vi "Wash - Activate LED.vi"(8 "error in (no error)":errorcluster, 11 "View Model":T2) -> (0 "error out":errorcluster, 2 "Wash LEDs":T1, 3 "View Model":T2)   [LabVIEW 2017]
doc: "Set active LED based on current wash step."
uses:
  View Model/Controls/View Model.ctl
  View Model/Controls/Shared Model.ctl
  Error Handler/Controls/Error Model.ctl
  Error Handler/Controls/Error Message.ctl
  Error Handler/Controls/Error Level.ctl
  Configuration/Controls/Database Model.ctl
  Configuration/Controls/Database Message.ctl
  Configuration/Controls/Database Command.ctl
  Configuration/Controls/Database Overhead.ctl
  Configuration/Controls/Database Status.ctl
  Configuration/Controls/Database Record.ctl
  Configuration/Controls/Database - Rule Record.ctl
  Controller/Controls/CNTRLR - Wash Step.ctl
  Controller/Controls/CNTRLR - Position.ctl
  Controller/Controls/CNTRLR - Model.ctl
  Controller/Controls/CNTRLR - Message.ctl
  Controller/Controls/CNTRLR - Command.ctl
  Controller/Controls/CNTRLR - Overhead.ctl
  Controller/Controls/CNTRLR - State.ctl
  Controls/Display - Wash LEDs.ctl
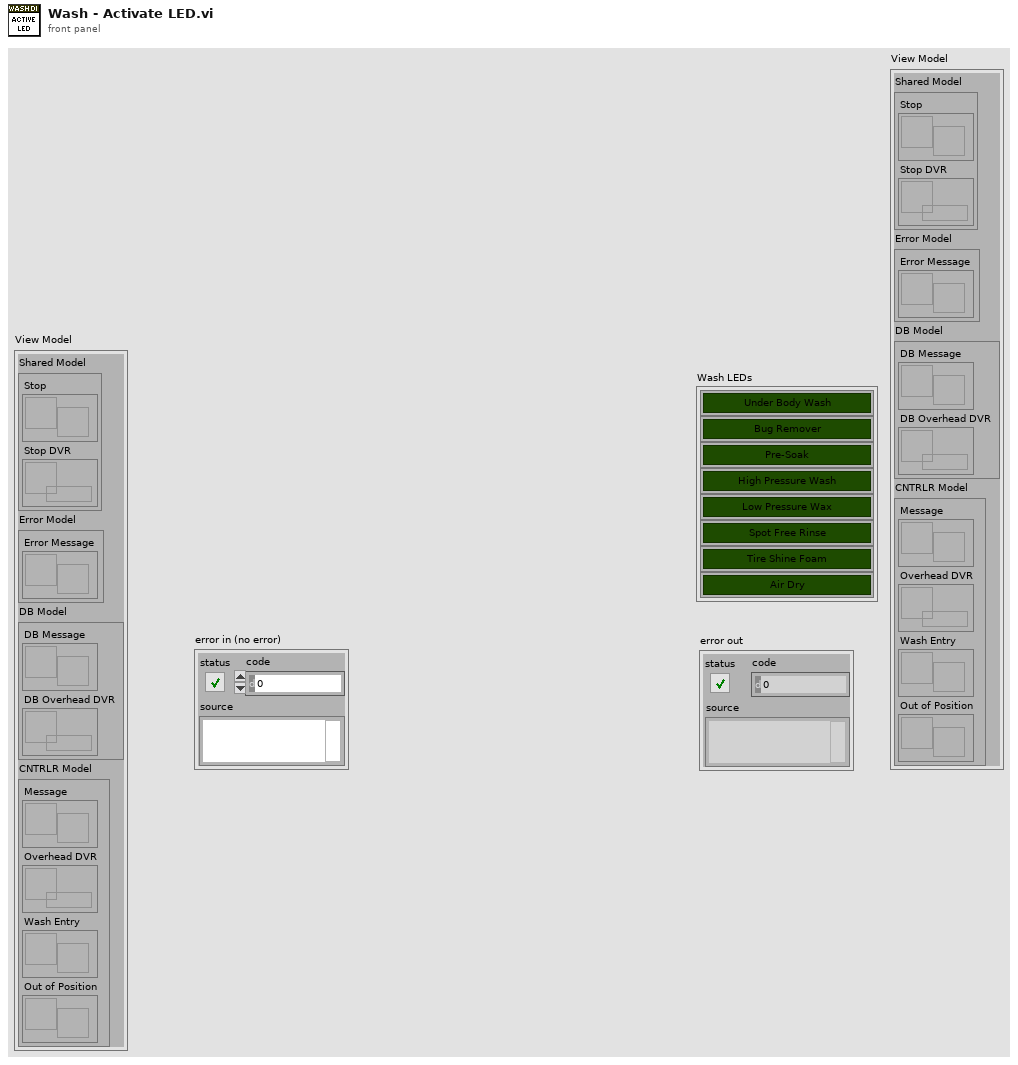
[diagram p1: front panel]
types:
  T1 = typedef "Display - Wash LEDs.ctl" = cluster{"Under Body Wash":bool, "Bug Remover":bool, "Pre-Soak":bool, "High Pressure Wash":bool, "Low Pressure Wax":bool, "Spot Free Rinse":bool, "Tire Shine Foam":bool, "Air Dry":bool}
  T2 = typedef "View Model.ctl" = cluster{"Shared Model":T3, "Error Model":T4, "DB Model":T5, "CNTRLR Model":T6}
  T3 = typedef "Shared Model.ctl" = cluster{"Stop":refnum<user-event>, "Stop DVR":refnum<data-value>}
  T4 = typedef "Error Model.ctl" = cluster{"Error Message":refnum<user-event>}
  T5 = typedef "Database Model.ctl" = cluster{"DB Message":refnum<user-event>, "DB Overhead DVR":refnum<data-value>}
  T6 = typedef "CNTRLR - Model.ctl" = cluster{"Message":refnum<user-event>, "Overhead DVR":refnum<data-value>, "Wash Entry":refnum<user-event>, "Out of Position":refnum<user-event>}
  T7 = typedef "CNTRLR - Wash Step.ctl" = enum16{"Under Body Wash", "Bug Remover", "Pre-Soak", "High Pressure Wash", "Low Pressure Wax", "Spot Free Rinse", "Tire Shine Foam", "Air Dry", "None"}
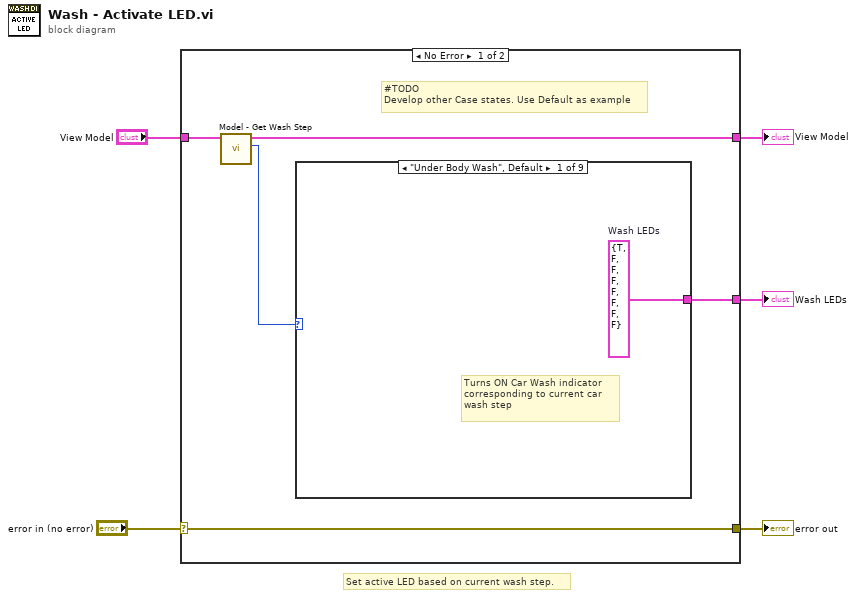
[diagram p0: block diagram]
diagram:
  # "Set active LED based on current wash step."
  n1 = case shown="No Error" "error in (no error)" {
    selector: "error in (no error)" -> [w10 w13]
    tunnel: [w10 w13] -> w4
    tunnel: "View Model" -> [w9 w12]
    tunnel: [w8 w12] -> w2
    tunnel: [w6 _] -> w1
    frame No Error {
      # "#TODO\nDevelop other Case states. Use Default as example"
      n2 = call "Model - Get Wash Step.vi"("View Model"=w9) -> ("Current Wash Step"=w7:T7, "View Model"=w8:T2)  [unwired: 8 in, 1 out]
      n3 = case shown="\"Under Body Wash\", Default" w7 {
        tunnel: [w11 _ _ _ _ _ _ _ _] -> w6
        frame "Under Body Wash", Default {
          w11 = T1 {"Under Body Wash"=TRUE, "Bug Remover"=FALSE, "Pre-Soak"=FALSE, "High Pressure Wash"=FALSE, "Low Pressure Wax"=FALSE, "Spot Free Rinse"=FALSE, "Tire Shine Foam"=FALSE, "Air Dry"=FALSE}  # Wash LEDs
          # "Turns ON Car Wash indicator\ncorresponding to current car \nwash step"
        }
        frame "Bug Remover" {
        }
        frame "Pre-Soak" {
        }
        frame "High Pressure Wash" {
        }
        frame "Low Pressure Wax" {
        }
        frame "Spot Free Rinse" {
        }
        frame "Tire Shine Foam" {
        }
        frame "Air Dry" {
        }
        frame "None" {
        }
      }
    }
    frame Error {
    }
  }
  "error out" <- w4
  "View Model" <- w2
  "Wash LEDs" <- w1
